vi "OAT Find Significant Orders.vi"(1 "num of significant orders":i32=5, 2 "order scale":cluster{"Offset":dbl, "Multiplier":dbl} {"Multiplier" format="%.2f"; "Offset" format="%.2f"}, 3 "order spectrum":dbl[][](array[numeric]) format="%.2f") -> (0 "orders":dbl[](array[numeric]) format="%.2f")   [LabVIEW 2017, in "SoundVib_Gabor.lvlib"]
uses:
  <vilib>/addons/Sound and Vibration/Order Analysis/Gabor Order Tracking/SoundVib_Gabor.lvlib
  <vilib>/Analysis/NI_AALBase.lvlib
  <vilib>/Analysis/NI_AALPro.lvlib
panel:
  in  "detect peak?":bool
  # "Find Significant Orders"
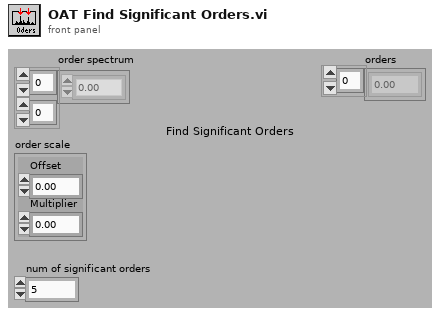
[diagram p1: front panel]
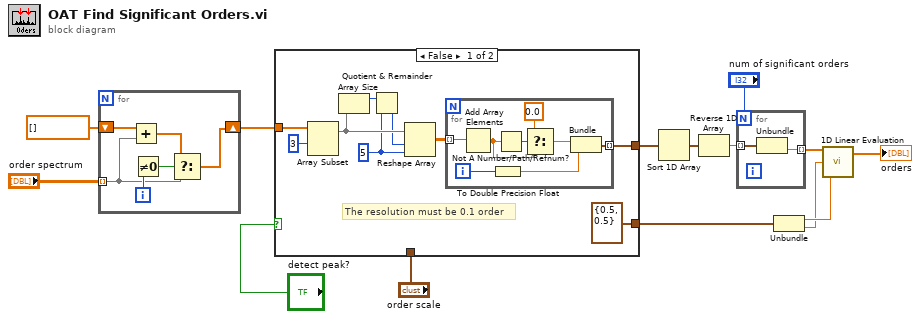
[diagram p0: block diagram]
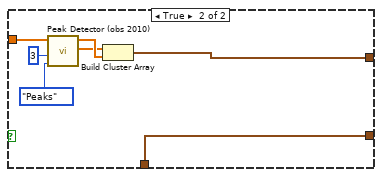
[diagram p2: hidden frame]
diagram:
  n1 = for {
    shift-right: [w16] -> w10
    shift-left: dbl[] [] -> [w18]
    tunnel: "order spectrum" -> [w15] mode=indexing
    i -> [w20]
    n2 = Add(x=w18, y=w15) -> (x+y=w17:dbl[])
    n3 = Not Equal To 0?(x=w20) -> (x != 0?=w19:bool)
    n4 = Select(t=w17, s=w19, f=w15) -> (s? t:f=w16:dbl[])
  }
  n5 = case shown="False" "detect peak?" {
    tunnel: [w22 w39] -> w1
    tunnel: w10 -> [w29 w42]
    tunnel: "order scale" -> [_ w38]
    tunnel: [cluster{"Offset":dbl, "Multiplier":dbl} {"Offset"=0.5, "Multiplier"=0.5} ("order scale") w38] -> w4
    frame False {
      w24 = 5 ("Dimension Size")
      # "The resolution must be 0.1 order"
      n6 = Array Subset(array=w29, index=3 ("Array Index")) -> (w26:dbl[])  [unwired: 1 in]
      n7 = Array Size(array=w26) -> (size(s)=w25:i32)
      n8 = Quotient & Remainder(x=w25, y=w24) -> (floor(x/y)=w23:i32)  [unwired: 1 out]
      n9 = Reshape Array(w26, w23, w24) -> (w27:dbl[][])
      n10 = for {
        tunnel: w27 -> [w37] mode=indexing
        tunnel: [w34] -> w22 mode=indexing
        i -> [w36]
        n11 = Add Array Elements(numeric array=w37) -> (sum=w30:dbl)
        n12 = To Double Precision Float(number=w36) -> (double precision float=w35:dbl)
        n13 = Not A Number/Path/Refnum?(number/path/refnum=w30) -> (NaN/Path/Refnum?=w33:bool)
        n14 = Select(t=0.0, s=w33, f=w30) -> (s? t:f=w32:dbl)
        n15 = Bundle("Numeric"=w32, w35) -> (w34:cluster{"Numeric":dbl, dbl})  [unwired: 1 in]
      }
    }
    frame True {
      n16 = call <vilib>:"Peak Detector (obs 2010).vi"("peaks/valleys"=enum32{"Peaks", "Valleys"}."Peaks", "width"=3, "X"=w42) -> ("Amplitudes"=w40:dbl[], "Locations"=w41:dbl[])  [unwired: 4 in, 3 out]
      n17 = Build Cluster Array(w40, w41) -> (w39:cluster{dbl, dbl}[])
    }
  }
  n18 = Sort 1D Array(array=w1) -> (sorted array=w7:cluster{"Numeric":dbl, dbl}[])
  n19 = Reverse 1D Array(array=w7) -> (reversed array=w9:cluster{"Numeric":dbl, dbl}[])
  n20 = for {
    N: "num of significant orders" -> [_]
    tunnel: w9 -> [w45] mode=indexing
    tunnel: [w46] -> w8 mode=indexing
    n21 = Unbundle(w45) -> (w46:dbl)  [unwired: 1 out]
  }
  n22 = Unbundle(w4) -> ("Offset"=w3:dbl, "Multiplier"=w2:dbl)
  n23 = call <vilib>:"1D Linear Evaluation.vi"("offset"=w3, "scale"=w2, "X"=w8) -> ("Y[i]=X[i]*a+b"=→"orders":dbl[])  [unwired: 1 out]
